vi "lib Version.vi"(8 "error in (no error)":errorcluster, 10 "version_size":u32, 11 "version":string) -> (0 "error out":errorcluster, 1 "function return":bool, 2 "version_size out":u32, 3 "version out":string)   [LabVIEW 2015, in "XGL_DPP.lvlib"]
doc: "EXTERN DECLSPEC bool CALL_CONV libVersion(char * version, uint32_t * version_size);"
uses:
  XGL_DPP.lvlib
  XGL_DPP.dll
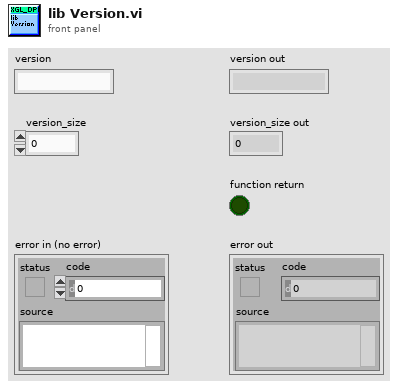
[diagram p1: front panel]
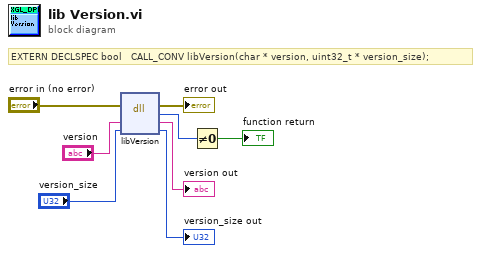
[diagram p0: block diagram]
diagram:
  # "EXTERN DECLSPEC bool   CALL_CONV libVersion(char * version, uint32_t * version_size);"
  n1 = dll-call lib="D:/Users/XRF/Desktop/Scanning Software_Demokritos_2015_v7/libs/Vis_2/XGL_DPP.*" fn="libVersion"(error in="error in (no error)", "version"="version", "version_size"="version_size") -> (error out=→"error out":errorcluster, w7:u8, "version"=→"version out":string, "version_size"=→"version_size out":u32)  [unwired: 2 in, 1 out]
  n2 = Not Equal To 0?(x=w7) -> (x != 0?=→"function return":bool)
